vi "PH_Beckhoff.get DE.vi"(0 "Digital Values":T1, 1 "index of element":i32) -> (2 "Value":bool, 3 "Quality":bool, 4 "Tag not found":bool)   [LabVIEW 2014, in "PH_Beckhoff.lvlib"]
uses:
  PH_Beckhoff.lvlib
  PH_Beckhoff.Digital Inputs.ctl
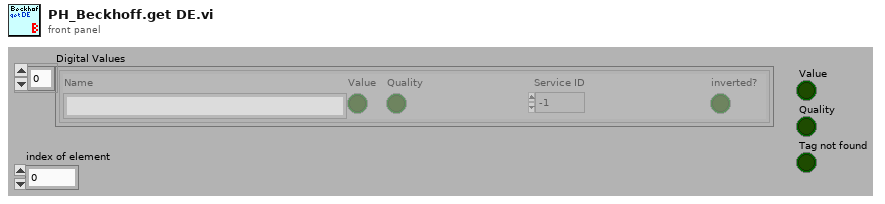
[diagram p1: front panel]
types:
  T1 = typedef "PH_Beckhoff.lvlib/PH_Beckhoff.Digital Inputs.ctl" = cluster{"Name":string, "Value":bool, "Quality":bool, "Service ID":i32, "inverted?":bool}[]
  T2 = cluster{"Name":string, "Value":bool, "Quality":bool, "Service ID":i32, "inverted?":bool}
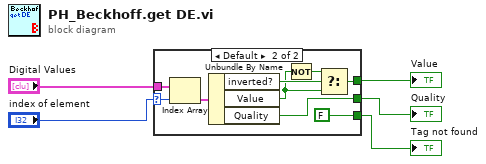
[diagram p0: block diagram]
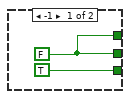
[diagram p2: hidden frame]
diagram:
  n1 = case shown="Default" "index of element" {
    selector: "index of element" -> [_ w14]
    tunnel: "Digital Values" -> [_ w16]
    tunnel: [w6 w13] -> w2
    tunnel: [TRUE FALSE] -> w4
    tunnel: [w6 w8] -> w5
    frame -1 {
      w6 = FALSE ("Quality")
    }
    frame Default {
      n2 = Index Array(array=w16, index=w14) -> (element=w15:T2)
      n3 = Unbundle By Name(w15) -> ("inverted?"=w11:bool, "Value"=w10:bool, "Quality"=w13:bool)
      n4 = Not(x=w10) -> (.not. x?=w9:bool)
      n5 = Select(t=w9, s=w11, f=w10) -> (s? t:f=w8:bool)
    }
  }
  "Value" <- w5
  "Tag not found" <- w4
  "Quality" <- w2
